vi "DataShow.vi"() -> (4 "数据":T1, 6 "Result":string[](array[string]), 10 "Status":string)   [LabVIEW 2015]
uses:
  2.ctl
panel:
  out "添加的数组":string[][](array[string])
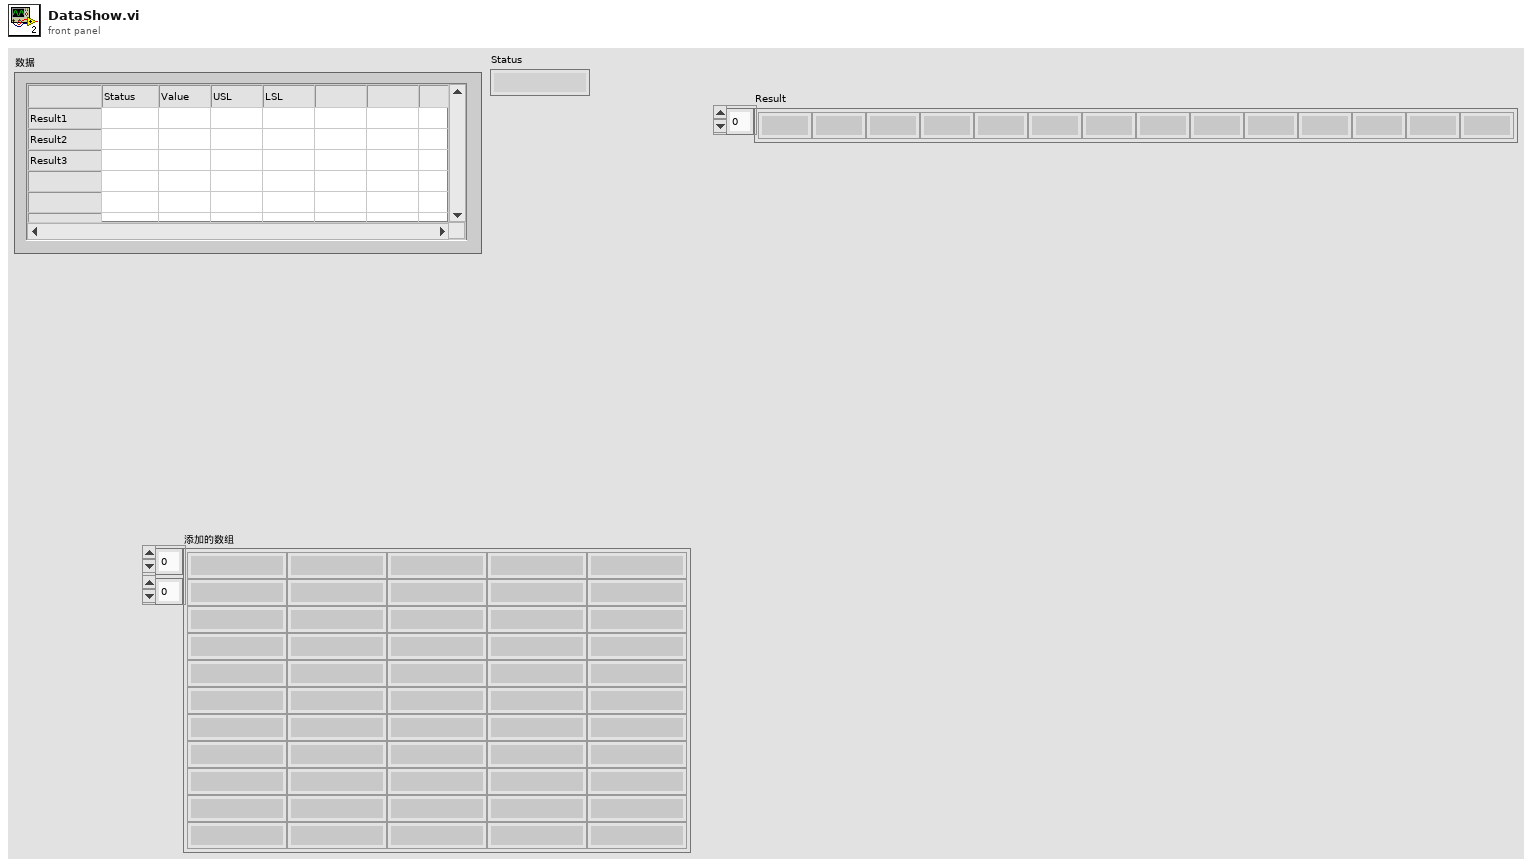
[diagram p1: front panel]
types:
  T1 = typedef "2.ctl" = string[][]
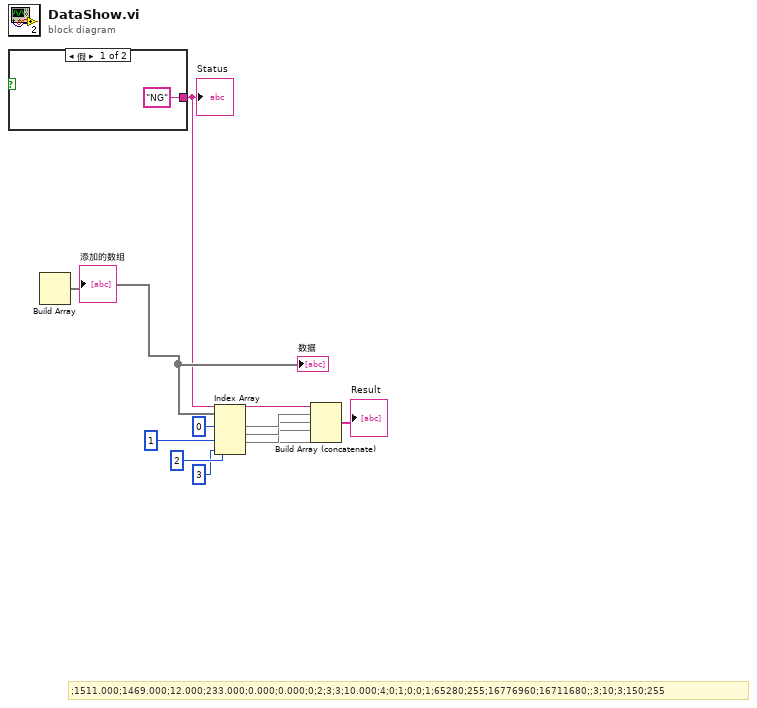
[diagram p0: block diagram]
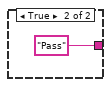
[diagram p2: hidden frame]
diagram:
  # ";1511.000;1469.000;12.000;233.000;0.000;0.000;0;2;3;3;10.000;4;0;1;0;0;1;65280;255;16776960;16711680;;3;10;3;150;255"
  n1 = case shown="假" w12 {
    tunnel: ["NG" "Pass"] -> w6
    frame False {
    }
    frame True {
    }
  }
  "Status" <- w6
  n2 = Build Array() -> (w11:void[], w13:dbl)  [unwired: 3 in]
  "数据" <- w11
  "添加的数组" <- w11
  n3 = Index Array(array=w11, index #1=0 ("索引 (行)"), index #2=1 ("索引 (行)"), index #3=2 ("索引 (行)"), index #4=3 ("索引 (行)")) -> (element #1=w7, element #2=w5, element #3=w4, element #4=w1)
  n4 = Build Array (concatenate)(w6, w7, w5, w4, w1) -> (→"Result":string[])
